vi "setCommandEvents.vi"(8 "error in (no error)":errorcluster, 10 "CommandEvents.lvclass":refnum<class "CommandEvents.lvclass">, 11 "SettingsViewer.lvclass in":refnum<class "settingsViewer.lvclass">) -> (0 "error out":errorcluster, 3 "SettingsViewer.lvclass out":refnum<class "settingsViewer.lvclass">)   [LabVIEW 2009, in "Views.lvlib" / "SettingsViewer.lvclass"]
uses:
  settingsViewer.lvclass
  CommandProcessor/CommandEvents/CommandEvents.lvclass
  settingsViewer.lvclass/settingsViewer.ctl
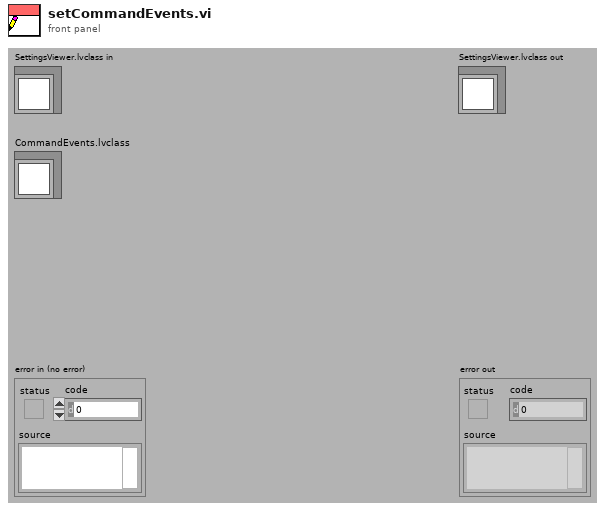
[diagram p1: front panel]
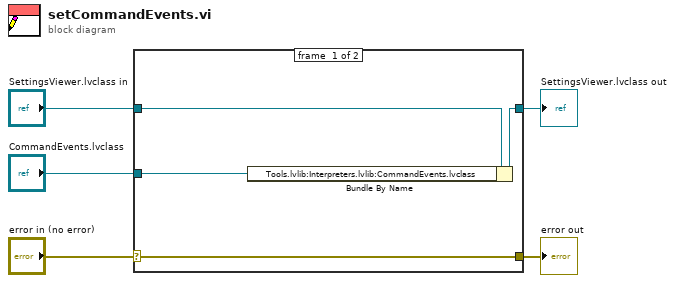
[diagram p0: block diagram]
diagram:
  n1 = case shown="No Error" "error in (no error)" {
    selector: "error in (no error)" -> [w9 w10]
    tunnel: [w9 w10] -> w4
    tunnel: [w7 w11] -> w2
    tunnel: "SettingsViewer.lvclass in" -> [w8 w11]
    tunnel: "CommandEvents.lvclass" -> [w6 _]
    frame #0 {
      n2 = Bundle By Name(cluster=w8, "Tools.lvlib:Interpreters.lvlib:CommandEvents.lvclass"=w6) -> (w7:refnum<class "settingsViewer.lvclass">)
    }
    frame #1 {
    }
  }
  "error out" <- w4
  "SettingsViewer.lvclass out" <- w2
